vi "Maxi Gauge-Channel-Sensor Identification.vi"(7 "W/R":bool, 8 "Fehler (Eingang, kein Fehler)":errorcluster caption="Fehler (Eingang)", 9 "Set Channel Identification":T1, 10 "Node address":i8=-1 min=-1 max=31 step=1, 11 "VISA-Ressource in":refnum<visa-resource-name>) -> (0 "Fehler (Ausgang)":errorcluster, 1 "Get Sensor Identification":T2, 2 "Get Channel Identification":T1, 3 "VISA-Ressource out":refnum<visa-resource-name>)   [LabVIEW 2013, in "Maxi Gauge.lvlib"]
uses:
  <instrlib>/Maxi Gauge/Maxi Gauge.lvlib
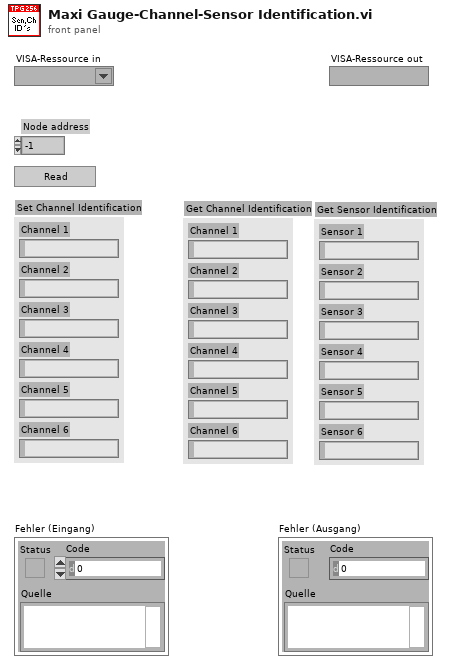
[diagram p1: front panel]
types:
  T1 = cluster{"Channel 1":string, "Channel 2":string, "Channel 3":string, "Channel 4":string, "Channel 5":string, "Channel 6":string}
  T2 = cluster{"Sensor 1":string, "Sensor 2":string, "Sensor 3":string, "Sensor 4":string, "Sensor 5":string, "Sensor 6":string}
  T3 = cluster{"[0]":string, "[1]":string, "[2]":string, "[3]":string, "[4]":string, "[5]":string}
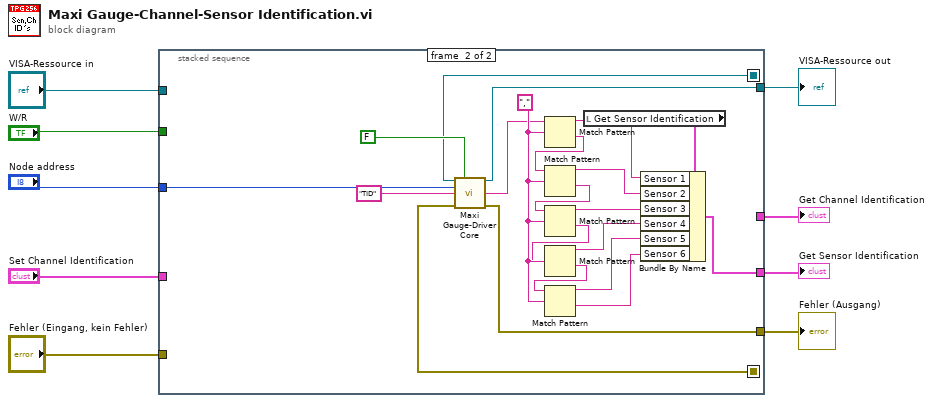
[diagram p0: block diagram]
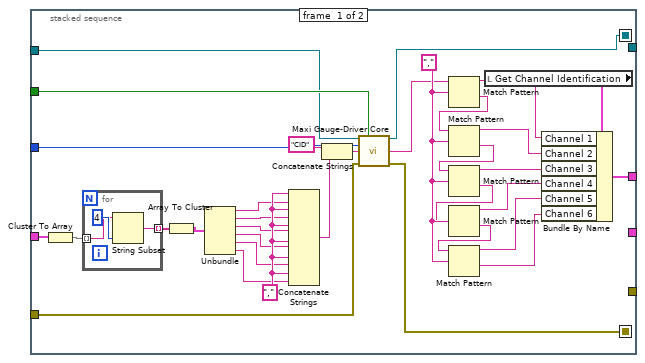
[diagram p2: hidden frame]
diagram:
  n1 = stacked-sequence {
    seq-local: [w12 _] -> [_ w50]
    seq-local: [w10 _] -> [_ w49]
    tunnel: "Node address" -> [w43 w67]
    tunnel: [w35 _] -> w8
    tunnel: [_ w52] -> w7
    tunnel: "W/R" -> [w28 _]
    tunnel: "Set Channel Identification" -> [w24 _]
    tunnel: "VISA-Ressource in" -> [w13 _]
    tunnel: "Fehler (Eingang, kein Fehler)" -> [w11 _]
    tunnel: [_ w48] -> w2
    tunnel: [_ w47] -> w1
    frame #0 {
      w25 = ","
      w42 = "," ("regular expression")
      n2 = Cluster To Array(cluster=w24) -> (array=w23:string[])
      n3 = for {
        tunnel: w23 -> [w45] mode=indexing
        tunnel: [w44] -> w22 mode=indexing
        n4 = String Subset(string=w45, length (rest)=4 ("length")) -> (substring=w44:string)  [unwired: 1 in]
      }
      n5 = Array To Cluster(array=w22) -> (cluster=w21:T3)
      n6 = Unbundle(w21) -> ("[0]"=w20:string, "[1]"=w19:string, "[2]"=w18:string, "[3]"=w17:string, "[4]"=w16:string, "[5]"=w15:string)
      n7 = Concatenate Strings(w25, w20, w25, w19, w25, w18, w25, w17, w25, w16, w25, w15) -> (w26:string)
      n8 = Concatenate Strings("CID" ("Command"), w26) -> (w14:string)
      n9 = call <instrlib>:"Maxi Gauge-Driver Core.vi"("VISA-Ressource in"=w13, "Write/Read"=w28, "Node address"=w43, "Command"=w14, "Fehler (Eingang)"=w11) -> ("VISA-Ressource out"=w12:refnum<visa-resource-name>, "String Out"=w41:string, "Fehler (Ausgang)"=w10:errorcluster)  [unwired: 8 in]
      n10 = Match Pattern(string=w41, regular expression=w42) -> (before substring=w34:string, after substring=w40:string)  [unwired: 1 in, 2 out]
      n11 = Match Pattern(string=w40, regular expression=w42) -> (before substring=w33:string, after substring=w39:string)  [unwired: 1 in, 2 out]
      n12 = Match Pattern(string=w39, regular expression=w42) -> (before substring=w32:string, after substring=w38:string)  [unwired: 1 in, 2 out]
      n13 = Match Pattern(string=w38, regular expression=w42) -> (before substring=w31:string, after substring=w37:string)  [unwired: 1 in, 2 out]
      n14 = Match Pattern(string=w37, regular expression=w42) -> (before substring=w30:string, after substring=w29:string)  [unwired: 1 in, 2 out]
      n15 = local read "Get Channel Identification"() -> (w36:T1)
      n16 = Bundle By Name(cluster=w36, "Channel 1"=w34, "Channel 2"=w33, "Channel 3"=w32, "Channel 4"=w31, "Channel 5"=w30, "Channel 6"=w29) -> (w35:T1)
    }
    frame #1 {
      w65 = "," ("regular expression")
      n17 = call <instrlib>:"Maxi Gauge-Driver Core.vi"("VISA-Ressource in"=w50, "Write/Read"=FALSE, "Node address"=w67, "Command"="TID", "Fehler (Eingang)"=w49) -> ("VISA-Ressource out"=w48:refnum<visa-resource-name>, "String Out"=w64:string, "Fehler (Ausgang)"=w47:errorcluster)  [unwired: 8 in]
      n18 = Match Pattern(string=w64, regular expression=w65) -> (before substring=w58:string, after substring=w63:string)  [unwired: 1 in, 2 out]
      n19 = Match Pattern(string=w63, regular expression=w65) -> (before substring=w57:string, after substring=w62:string)  [unwired: 1 in, 2 out]
      n20 = Match Pattern(string=w62, regular expression=w65) -> (before substring=w56:string, after substring=w61:string)  [unwired: 1 in, 2 out]
      n21 = Match Pattern(string=w61, regular expression=w65) -> (before substring=w55:string, after substring=w60:string)  [unwired: 1 in, 2 out]
      n22 = Match Pattern(string=w60, regular expression=w65) -> (before substring=w54:string, after substring=w53:string)  [unwired: 1 in, 2 out]
      n23 = local read "Get Sensor Identification"() -> (w59:T2)
      n24 = Bundle By Name(cluster=w59, "Sensor 1"=w58, "Sensor 2"=w57, "Sensor 3"=w56, "Sensor 4"=w55, "Sensor 5"=w54, "Sensor 6"=w53) -> (w52:T2)
    }
  }
  "Get Channel Identification" <- w8
  "Get Sensor Identification" <- w7
  "VISA-Ressource out" <- w2
  "Fehler (Ausgang)" <- w1
